vi "point clicked on graph.vi"(9 "Mouse Position":T1, 11 "Graphchart reference":refnum<vi>) -> (1 "Point clicked":cluster{"x":dbl, "y":dbl}, 2 "Valid mouse position":bool)   [LabVIEW 2009]
uses:
  <vilib>/Utility/miscctls.llb/LVPoint32TypeDef.ctl
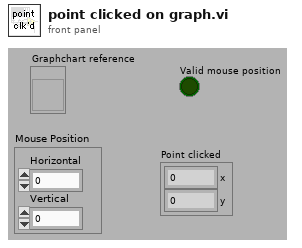
[diagram p1: front panel]
types:
  T1 = typedef "LVPoint32TypeDef.ctl" = cluster{"Horizontal":i32, "Vertical":i32}
  T2 = typedef "LVRectTypeDef.ctl" = cluster{"left":i16, "top":i16, "right":i16, "bottom":i16}
  T3 = typedef "LVBoundsTypeDef.ctl" = cluster{"Width":u32, "Height":u32}
  T4 = cluster{"XScale.Maximum":dbl, "YScale.Minimum":dbl}
  T5 = cluster{"XScale.Minimum":dbl, "YScale.Maximum":dbl}
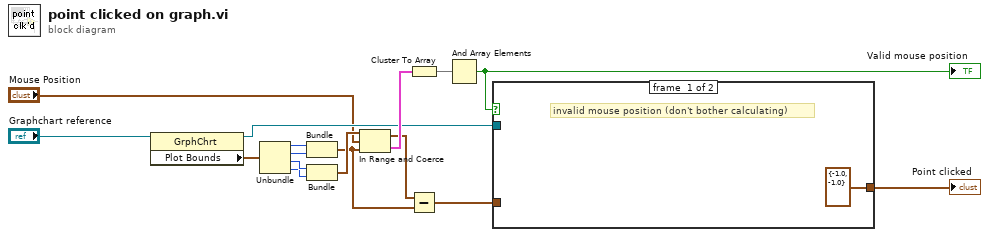
[diagram p0: block diagram]
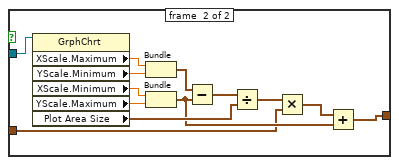
[diagram p2: hidden frame]
diagram:
  n1 = property on="Property Node" class="GrphChrt"(reference="Graphchart reference") -> (reference out=w6:refnum<vi>, "Plot Bounds"=w8:T2)  [unwired: 1 in, 1 out]
  n2 = Unbundle(w8) -> ("left"=w15:i16, "top"=w14:i16, "right"=w13:i16, "bottom"=w12:i16)
  n3 = Bundle("left"=w15, "top"=w14) -> (w1:cluster{"left":i16, "top":i16})  [unwired: 1 out]
  n4 = Bundle("right"=w13, "bottom"=w12) -> (w11:cluster{"right":i16, "bottom":i16})  [unwired: 1 out]
  n5 = In Range and Coerce(upper limit=w11, x="Mouse Position", lower limit=w1) -> (coerced(x)=w5:T1, In Range?=w10:cluster{"Horizontal":bool, "Vertical":bool})
  n6 = Cluster To Array(cluster=w10) -> (array=w9:bool[])
  n7 = Subtract(x=w5, y=w1) -> (x-y=w2:T1)
  n8 = And Array Elements(Boolean array=w9) -> (logical AND=w7:bool)
  "Valid mouse position" <- w7
  n9 = case shown="True" w7 {
    tunnel: w6 -> [_ w30]
    tunnel: w2 -> [_ w18]
    tunnel: [cluster{dbl, dbl} {-1.0, -1.0} w28] -> w4
    frame #0 {
      # "invalid mouse position (don't bother calculating)"
    }
    frame #1 {
      n10 = property on="Property Node" class="GrphChrt"(reference=w30) -> ("XScale.Maximum"=w27:dbl, "YScale.Minimum"=w26:dbl, "XScale.Minimum"=w25:dbl, "YScale.Maximum"=w24:dbl, "Plot Area Size"=w21:T3)  [unwired: 1 in, 2 out]
      n11 = Bundle("XScale.Maximum"=w27, "YScale.Minimum"=w26) -> (w23:T4)  [unwired: 1 out]
      n12 = Bundle("XScale.Minimum"=w25, "YScale.Maximum"=w24) -> (w20:T5)  [unwired: 1 out]
      n13 = Subtract(x=w23, y=w20) -> (x-y=w22:cluster{dbl, dbl})
      n14 = Divide(x=w22, y=w21) -> (x/y=w19:cluster{dbl, dbl})
      n15 = Multiply(x=w19, y=w18) -> (x*y=w29:cluster{dbl, dbl})
      n16 = Add(x=w29, y=w20) -> (x+y=w28:cluster{dbl, dbl})
    }
  }
  "Point clicked" <- w4
